vi "Get Field Types.vi"(8 "error in (no error)":errorcluster, 11 "Basic Form in":refnum<class "Basic Form.lvclass">) -> (0 "error out":errorcluster, 3 "Basic Form out":refnum<class "Basic Form.lvclass">)   [LabVIEW 2020, in "Form.lvlib" / "Basic Form.lvclass"]
uses:
  Basic Form.lvclass
  C:/Users/User/Desktop/Raman Program/Database OOP/source/Database OOP/Table Libraries/Basic Table/Basic Table Class/Basic Table.lvclass
  Basic Table/Basic Table Class/Basic Table.lvclass/Basic Table.ctl
  Basic Form.lvclass/Basic Form.ctl
  Column Libraries/Column Interface/Column Interface Class/Column Interface.lvclass
  Basic Table/Basic Table Class/Basic Table.lvclass
panel:
  out "Field Types":map{string, string}(c390)
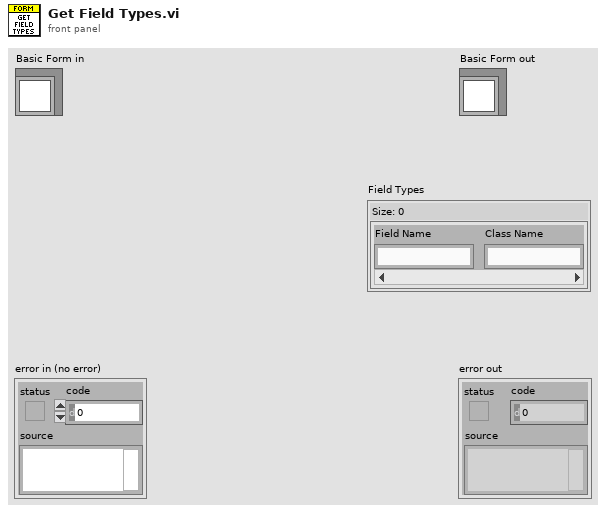
[diagram p1: front panel]
types:
  T1 = map{string, refnum<class "Column Interface.lvclass">}
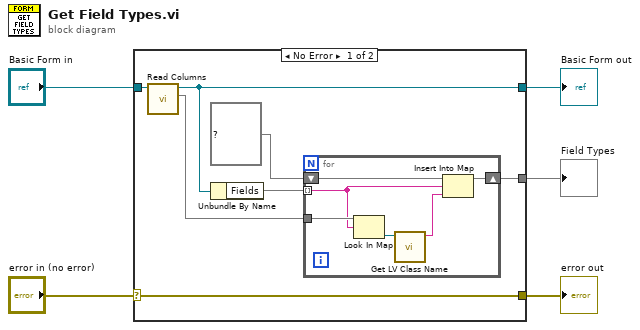
[diagram p0: block diagram]
diagram:
  n1 = case shown="No Error" "error in (no error)" {
    selector: "error in (no error)" -> [w12 w20]
    tunnel: [w12 w20] -> w4
    tunnel: [w9 w19] -> w2
    tunnel: "Basic Form in" -> [w10 w19]
    tunnel: [w6 _] -> w1
    frame No Error {
      n2 = call "Read Columns.vi"("Basic Table in"=w10) -> ("Columns"=w8:T1, "Basic Table out"=w9:refnum<class "Basic Form.lvclass">)  [unwired: 8 in, 1 out]
      n3 = Unbundle By Name(w9) -> ("Fields"=w11:set{string})
      n4 = for {
        tunnel: w11 -> [w15] mode=indexing
        tunnel: w8 -> [w18]
        shift-right: [w13] -> w6
        shift-left: map{string, string} {} ("Field Types") -> [w14]
        n5 = Look In Map(map=w18, key=w15) -> (value=w17:refnum<class "Column Interface.lvclass">)  [unwired: 1 in, 1 out]
        n6 = call <vilib>:"Get LV Class Name.vi"("object"=w17) -> ("class name"=w16:string)  [unwired: 9 in, 1 out]
        n7 = Insert Into Map(map in=w14, key=w15, value=w16) -> (map out=w13:map{string, string})  [unwired: 2 out]
      }
    }
    frame Error {
    }
  }
  "error out" <- w4
  "Basic Form out" <- w2
  "Field Types" <- w1
